vi "Video Processing.vi"() -> ()   [LabVIEW 2016]
uses:
  <vilib>/vision/driver/NI_Vision_Acquisition_Software.lvlib
  <vilib>/vision/NI_Vision_Development_Module.lvlib
panel:
  in  "Erode Number of iterations (1)":i32=1
  out "Degrees to turn":dbl
  out "Turn Direction":string
  out "abs(x)":dbl
  out "Hook found":bool
  out "Turn left/right":bool
  out "Hook-robot":dbl
  out "Center":dbl
  out "x/y":dbl
  out "Particle Measurements (Pixels)":dbl[][](array[numeric]) format="%.2f"
  in  "Pixel Measurements 2":T1[](array[typedef]) items=["Center of Mass X", "Center of Mass Y", "First Pixel X", "First Pixel Y", "Bounding Rect Left", "Bounding Rect Top", "Bounding Rect Right", "Bounding Rect Bottom", "Max Feret Diameter Start X", "Max Feret Diameter Start Y", "Max Feret Diameter End X", "Max Feret Diameter End Y", "Max Horiz. Segment Length Left", "Max Horiz. Segment Length Right", "Max Horiz. Segment Length Row", "-", "Bounding Rect Width", "Bounding Rect Height", "Bounding Rect Diagonal", "Perimeter", "Convex Hull Perimeter", "Holes' Perimeter", "Max Feret Diameter", "Equivalent Ellipse Major Axis", "Equivalent Ellipse Minor Axis", "Equivalent Ellipse Minor Axis (Feret)", "Equivalent Rect Long Side", "Equivalent Rect Short Side", "Equivalent Rect Diagonal", "Equivalent Rect Short Side (Feret)", "Average Horiz. Segment Length", "Average Vert. Segment Length", "Hydraulic Radius", "Waddel Disk Diameter", "-", "Area", "Holes' Area", "Particle & Holes' Area", "Convex Hull Area", "Image Area", "-", "Number of Holes", "Number of Horiz. Segments", "Number of Vert. Segments", "-", "Orientation", "Max Feret Diameter Orientation", "-", "% Area/Image Area", "% Area/(Particle & Holes' Area)", "Ratio of Equivalent Ellipse Axes", "Ratio of Equivalent Rect Sides", "-", "Elongation Factor", "Compactness Factor", "Heywood Circularity Factor", "Type Factor", "-", "Sum X", "Sum Y", "Sum XX", "Sum XY", "Sum YY", "Sum XXX", "Sum XXY", "Sum XYY", "Sum YYY", "-", "Moment of Inertia XX", "Moment of Inertia XY", "Moment of Inertia YY", "Moment of Inertia XXX", "Moment of Inertia XXY", "Moment of Inertia XYY", "Moment of Inertia YYY", "Norm. Moment of Inertia XX", "Norm. Moment of Inertia XY", "Norm. Moment of Inertia YY", "Norm. Moment of Inertia XXX", "Norm. Moment of Inertia XXY", "Norm. Moment of Inertia XYY", "Norm. Moment of Inertia YYY", "Hu Moment 1", "Hu Moment 2", "Hu Moment 3", "Hu Moment 4", "Hu Moment 5", "Hu Moment 6", "Hu Moment 7"]
  out "subarray":dbl[](array[numeric])
  out "Sorted Data":dbl[][](array[numeric])
  out "Particles":i32
  in  "Min Area Size %":dbl
  in  "Pixel Measurements":T1[](array[typedef])=[35, 4, 5, 6, 7] items=["Center of Mass X", "Center of Mass Y", "First Pixel X", "First Pixel Y", "Bounding Rect Left", "Bounding Rect Top", "Bounding Rect Right", "Bounding Rect Bottom", "Max Feret Diameter Start X", "Max Feret Diameter Start Y", "Max Feret Diameter End X", "Max Feret Diameter End Y", "Max Horiz. Segment Length Left", "Max Horiz. Segment Length Right", "Max Horiz. Segment Length Row", "-", "Bounding Rect Width", "Bounding Rect Height", "Bounding Rect Diagonal", "Perimeter", "Convex Hull Perimeter", "Holes' Perimeter", "Max Feret Diameter", "Equivalent Ellipse Major Axis", "Equivalent Ellipse Minor Axis", "Equivalent Ellipse Minor Axis (Feret)", "Equivalent Rect Long Side", "Equivalent Rect Short Side", "Equivalent Rect Diagonal", "Equivalent Rect Short Side (Feret)", "Average Horiz. Segment Length", "Average Vert. Segment Length", "Hydraulic Radius", "Waddel Disk Diameter", "-", "Area", "Holes' Area", "Particle & Holes' Area", "Convex Hull Area", "Image Area", "-", "Number of Holes", "Number of Horiz. Segments", "Number of Vert. Segments", "-", "Orientation", "Max Feret Diameter Orientation", "-", "% Area/Image Area", "% Area/(Particle & Holes' Area)", "Ratio of Equivalent Ellipse Axes", "Ratio of Equivalent Rect Sides", "-", "Elongation Factor", "Compactness Factor", "Heywood Circularity Factor", "Type Factor", "-", "Sum X", "Sum Y", "Sum XX", "Sum XY", "Sum YY", "Sum XXX", "Sum XXY", "Sum XYY", "Sum YYY", "-", "Moment of Inertia XX", "Moment of Inertia XY", "Moment of Inertia YY", "Moment of Inertia XXX", "Moment of Inertia XXY", "Moment of Inertia XYY", "Moment of Inertia YYY", "Norm. Moment of Inertia XX", "Norm. Moment of Inertia XY", "Norm. Moment of Inertia YY", "Norm. Moment of Inertia XXX", "Norm. Moment of Inertia XXY", "Norm. Moment of Inertia XYY", "Norm. Moment of Inertia YYY", "Hu Moment 1", "Hu Moment 2", "Hu Moment 3", "Hu Moment 4", "Hu Moment 5", "Hu Moment 6", "Hu Moment 7"]
  in  "Particle Count Limit":dbl=2.0 format="%#_13g"
  out "Image 4":T2(plugin-control)
  out "error out":errorcluster
  in  "Range":cluster{"Lower value":sgl, "Upper value":sgl}={"Lower value"=128.0, "Upper value"=255.0} {"Upper value" format="%.2f"; "Lower value" format="%.2f"}
  in  "Color Plane":i32(ring)=1 items=["Red", "Green", "Blue", "Hue", "Saturation", "Luminance", "Value", "Intensity"]
  in  "Camera Name":refnum<k21>="cam1" caption="IMAQdx Session"
  in  "Stop":bool
  out "Frame Rate":dbl(knob) scale=0.0..100.0
  out "Image":T2(plugin-control)
  out "Buffer Number":u32
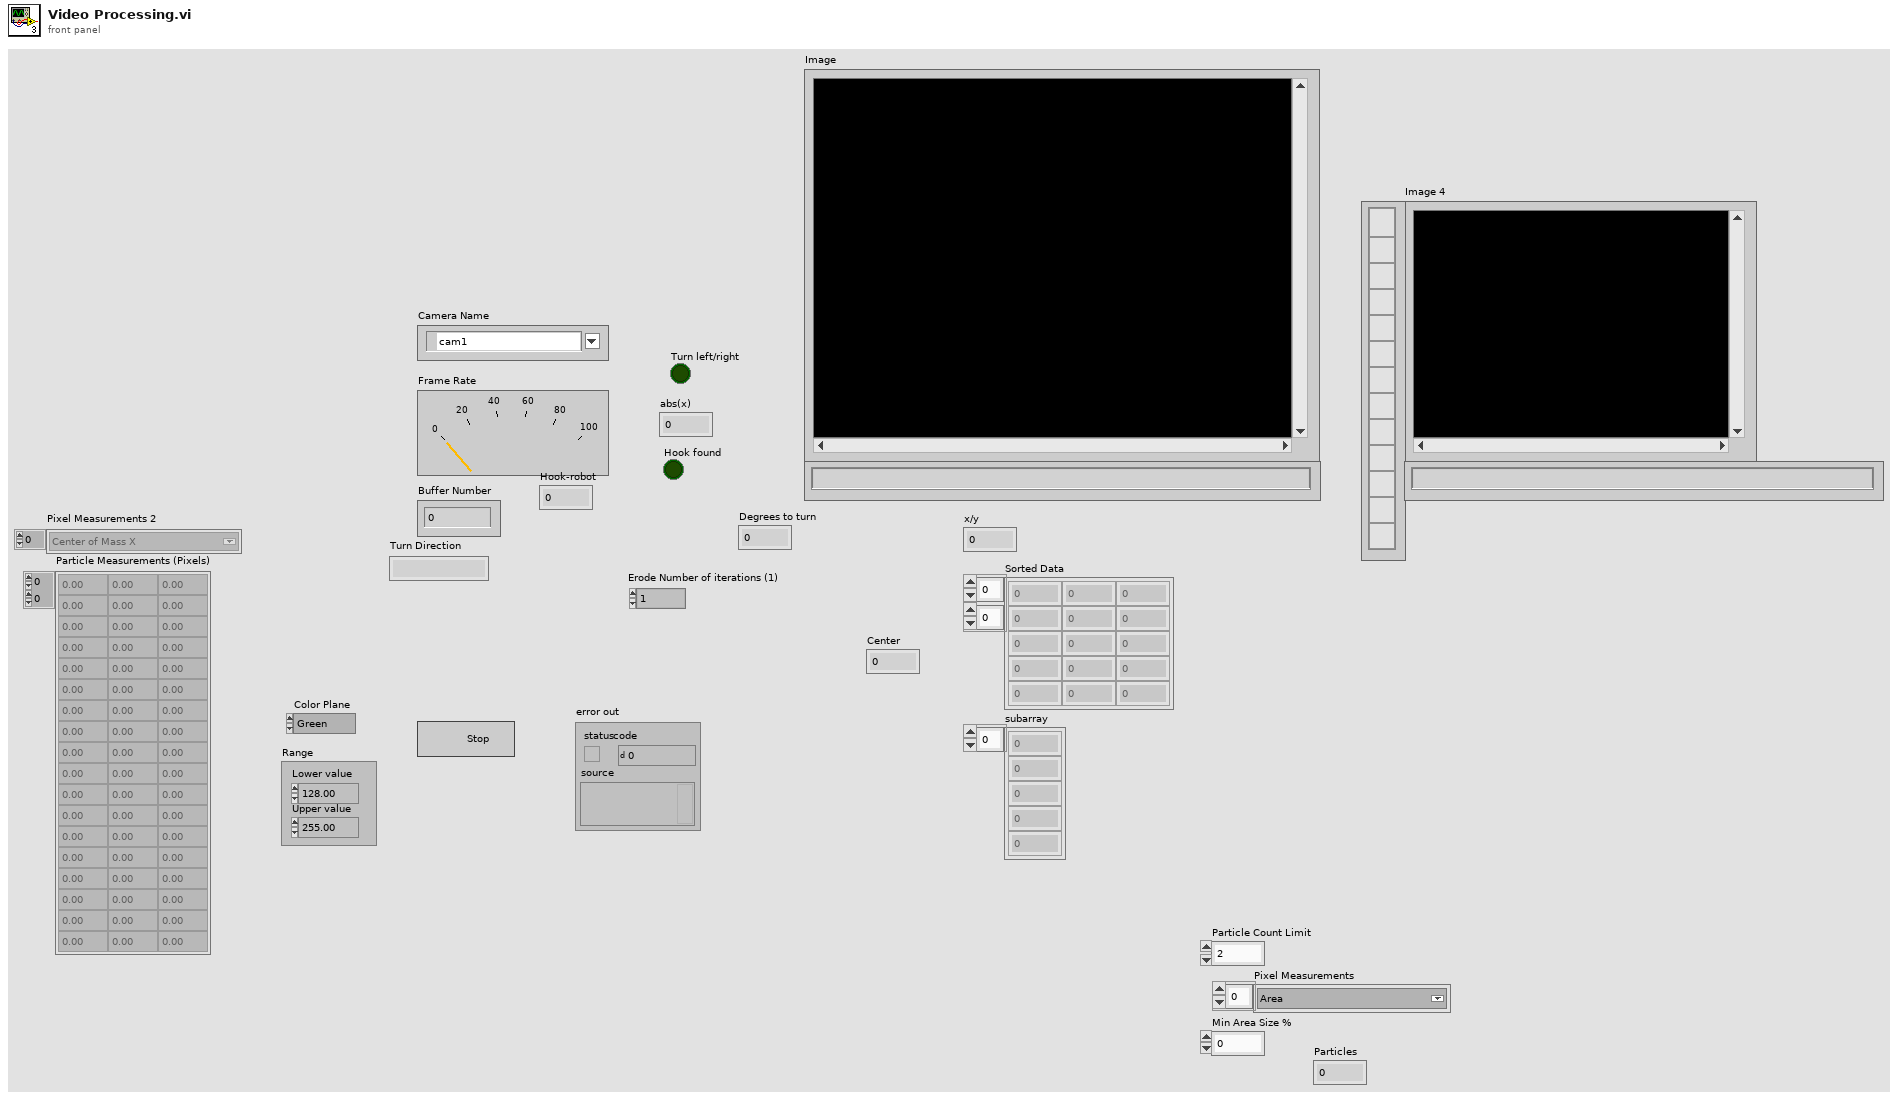
[diagram p1: front panel]
types:
  T1 = typedef "Particle Parameters" = i32
  T2 = typedef "IMAQ Image.ctl" = refnum<image>
  T3 = typedef "Image Type" = u32
  T4 = typedef "IMAQdx.ctl" = refnum<k21>
  T5 = enum32{"AutoM", "Close", "Dilate", "Erode", "Gradient", "Gradient in", "Gradient out", "HitMiss", "Open", "PClose", "POpen", "Thick", "Thin"}
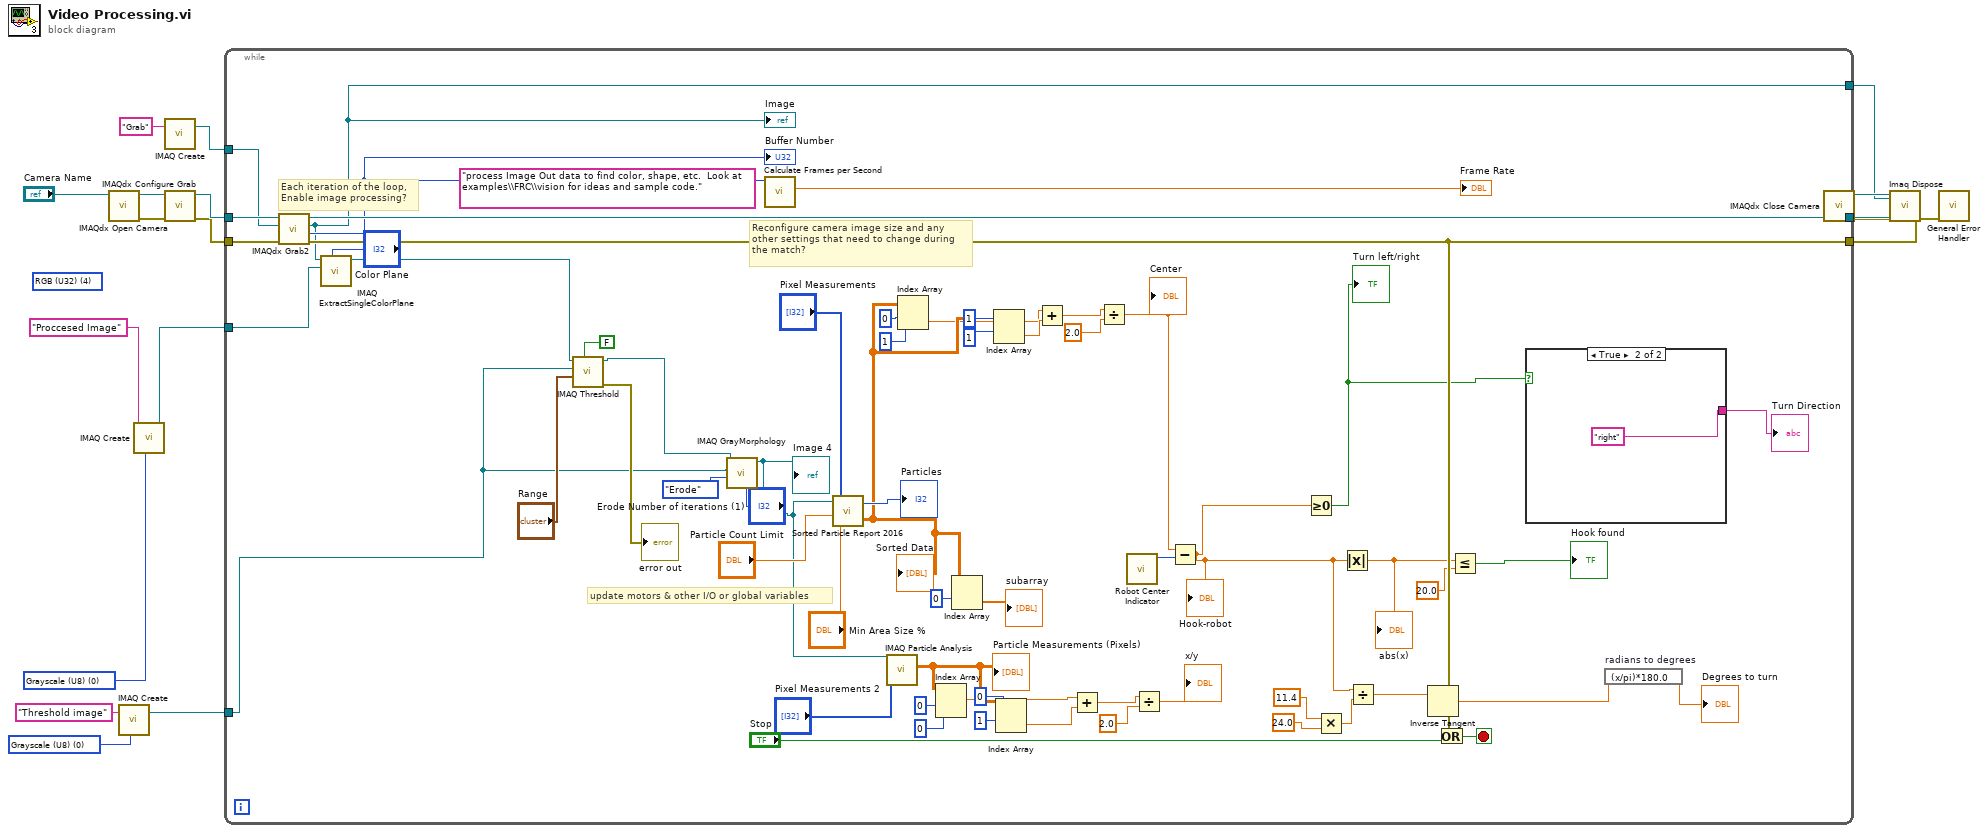
[diagram p0: block diagram]
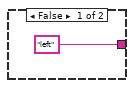
[diagram p2: hidden frame]
diagram:
  w3 = T3 0 items=["Grayscale (U8)", "Grayscale (I16)", "Grayscale (SGL)", "Complex (CSG)", "RGB (U32)", "HSL (U32)", "RGB (U64)"] ("Image Type")
  w5 = T3 0 items=["Grayscale (U8)", "Grayscale (I16)", "Grayscale (SGL)", "Complex (CSG)", "RGB (U32)", "HSL (U32)", "RGB (U64)"] ("Image Type")
  (unwired) T3 4 items=["Grayscale (U8)", "Grayscale (I16)", "Grayscale (SGL)", "Complex (CSG)", "RGB (U32)", "HSL (U32)", "RGB (U64)"] ("Image Type")
  n1 = call <vilib>:"IMAQdx Open Camera.vi"("Session In"="Camera Name") -> ("error out"=w13:errorcluster, "Session Out"=w12:T4)  [unwired: 2 in, 7 out]
  n2 = call "IMAQ Create"("Image Name"="Threshold image", "Image Type"=w3) -> ("New Image"=w1:T2)  [unwired: 2 in, 2 out]
  n3 = call "IMAQ Create"("Image Name"="Proccesed Image", "Image Type"=w5) -> ("New Image"=w2:T2)  [unwired: 2 in, 2 out]
  n4 = call "IMAQ Create"("Image Name"="Grab") -> ("New Image"=w18:T2)  [unwired: 3 in, 2 out]
  n5 = call <vilib>:"IMAQdx Configure Grab.vi"("error in"=w13, "Session In"=w12) -> ("error out"=w16:errorcluster, "Session Out"=w17:T4)  [unwired: 8 out]
  n6 = while {
    tunnel: [w74] -> w15
    tunnel: w16 -> [w76]
    tunnel: w17 -> [w77]
    tunnel: [w71] -> w14
    tunnel: w18 -> [w75]
    tunnel: [w25] -> w10
    tunnel: w2 -> [w24]
    tunnel: w1 -> [w21]
    stop <- w79 stop-if-true
    (unwired) "process Image Out data to find color, shape, etc.  Look at examples\\FRC\\vision for ideas and sample code."
    # "update motors & other I/O or global variables"
    # "Reconfigure camera image size and any\nother settings that need to change during\nthe match?"
    # "Each iteration of the loop,\nEnable image processing?"
    n7 = call <vilib>:"IMAQdx Grab2.vi"("error in"=w76, "Image In"=w75, "Session In"=w77) -> ("error out"=w71:errorcluster, "Buffer Number Out"=w72:u32, "Image Out"=w25:T2, "Session Out"=w74:T4)  [unwired: 5 in]
    "Image" <- w25
    "Buffer Number" <- w72
    n8 = call "IMAQ ExtractSingleColorPlane"("Color Plane"="Color Plane", "Image Dst"=w24, "Image Src"=w25) -> ("Image Dst Out"=w69:T2)  [unwired: 7 in, 1 out]
    n9 = call "IMAQ Threshold"("Keep/Replace Value (Replace)"=FALSE, "Range"="Range", "Image Dst"=w21, "Image Src"=w69) -> ("error out"=→"error out":errorcluster, "Image Dst Out"=w22:T2)  [unwired: 6 in]
    n10 = call "IMAQ GrayMorphology"("Number of iterations (1)"="Erode Number of iterations (1)", "Operation"=T5."Erode", "Image Dst"=w21, "Image Src"=w22) -> ("Image Dst Out"=w20:T2)  [unwired: 6 in, 1 out]
    "Image 4" <- w20
    n11 = call <vilib>:"Calculate Frames per Second.vi"("Buffer Number"=w72) -> ("Processed Frames/s"=→"Frame Rate":dbl)  [unwired: 8 in, 2 out]
    n12 = call "Sorted Particle Report 2016.vi"("Min Area Size %"="Min Area Size %", "Particle Count Limit"="Particle Count Limit", "Pixel Measurements"="Pixel Measurements", "Image in"=w20) -> ("Sorted Data"=w45:dbl[][], "Particles"=→"Particles":i32)
    "Sorted Data" <- w45
    n13 = call "IMAQ Particle Analysis"("Pixel Measurements"="Pixel Measurements 2", "Image"=w20) -> ("Particle Measurements (Pixels)"=w57:dbl[][])  [unwired: 3 in, 6 out]
    "Particle Measurements (Pixels)" <- w57
    n14 = Index Array(array=w45, index (row)=0, index (col)=1 ("disabled index (col)")) -> (element=w43:dbl)
    n15 = Index Array(array=w57, index (row)=0, index (col)=0 ("disabled index (col)")) -> (element=w55:dbl)
    n16 = Index Array(array=w45, index (row)=0) -> (element=→"subarray":dbl[])  [unwired: 1 in]
    n17 = Index Array(array=w45, index (row)=1, index (col)=1 ("disabled index (col)")) -> (element=w44:dbl)
    n18 = Index Array(array=w57, index (row)=1, index (col)=0 ("disabled index (col)")) -> (element=w54:dbl)
    n19 = Add(x=w43, y=w44) -> (x+y=w47:dbl)
    n20 = Add(x=w55, y=w54) -> (x+y=w53:dbl)
    n21 = Divide(x=w47, y=2.0) -> (x/y=w36:dbl)
    "Center" <- w36
    n22 = call "Robot Center Indicator.vi"() -> ("Robot Center"=w39:i32)  [unwired: 10 in, 1 out]
    n23 = Divide(x=w53, y=2.0) -> (x/y=→"x/y":dbl)
    n24 = Subtract(x=w36, y=w39) -> (x-y=w32:dbl)
    "Hook-robot" <- w32
    n25 = Greater Or Equal To 0?(x=w32) -> (x >= 0?=w34:bool)
    "Turn left/right" <- w34
    n26 = Multiply(x=11.4, y=24.0) -> (x*y=w29:dbl)
    n27 = Absolute Value(x=w32) -> (abs(x)=w38:dbl)
    "abs(x)" <- w38
    n28 = Divide(x=w32, y=w29) -> (x/y=w28:dbl)
    n29 = Inverse Tangent(1:w28) -> (0:w27:dbl)
    n30 = Or(x=w71, y="Stop") -> (x .or. y?=w79:bool)
    n31 = Less Or Equal?(x=w38, y=20.0) -> (x <= y?=→"Hook found":bool)
    n32 = case shown="True" w34 {
      tunnel: ["left" ("Turn Direction") "right" ("Turn Direction")] -> w33
      frame False {
      }
      frame True {
      }
    }
    "Turn Direction" <- w33
    n33 = expression code="(x/pi)*180.0" "radians to degrees"(w27) -> (→"Degrees to turn":dbl)
  }
  n34 = call <vilib>:"IMAQdx Close Camera.vi"("error in"=w14, "Session In"=w15) -> ("error out"=w9:errorcluster)  [unwired: 9 out]
  n35 = call "Imaq Dispose"("Image"=w10, "error in (no error)"=w9) -> ("error out"=w8:errorcluster)  [unwired: 4 in]
  n36 = call <vilib>:"General Error Handler.vi"("error in (no error)"=w8) -> ()  [unwired: 2 in, 13 out]
